vi "HRV_뽑아내기.vi"() -> ()   [LabVIEW 2014]
uses:
  <vilib>/Utility/file.llb/Read From Spreadsheet File (string).vi
  <vilib>/Utility/file.llb/Read From Spreadsheet File (I64).vi
  <vilib>/Utility/file.llb/Read From Spreadsheet File (DBL).vi
  <vilib>/Utility/file.llb/Write To Spreadsheet File (DBL).vi
panel:
  out "Array":dbl[][](array[numeric])
  in  "피험자이름":path=path "C:/Users/Jaehong/Desktop/Classifiers/HRV_EEG/ERP_total/강병훈/ERP_total.txt"
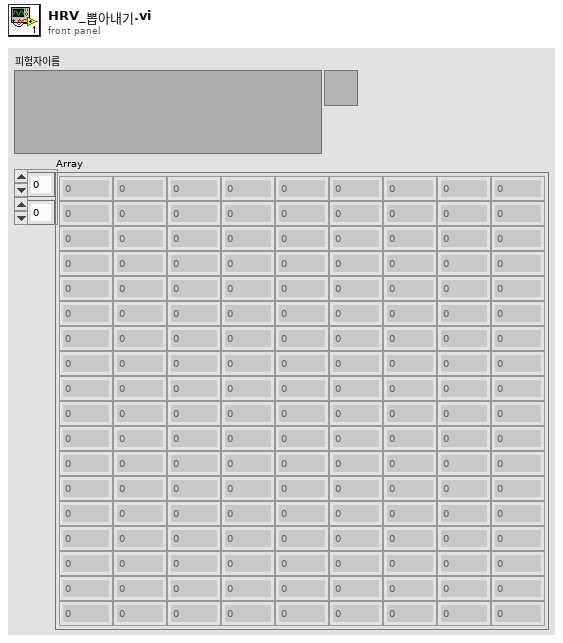
[diagram p1: front panel]
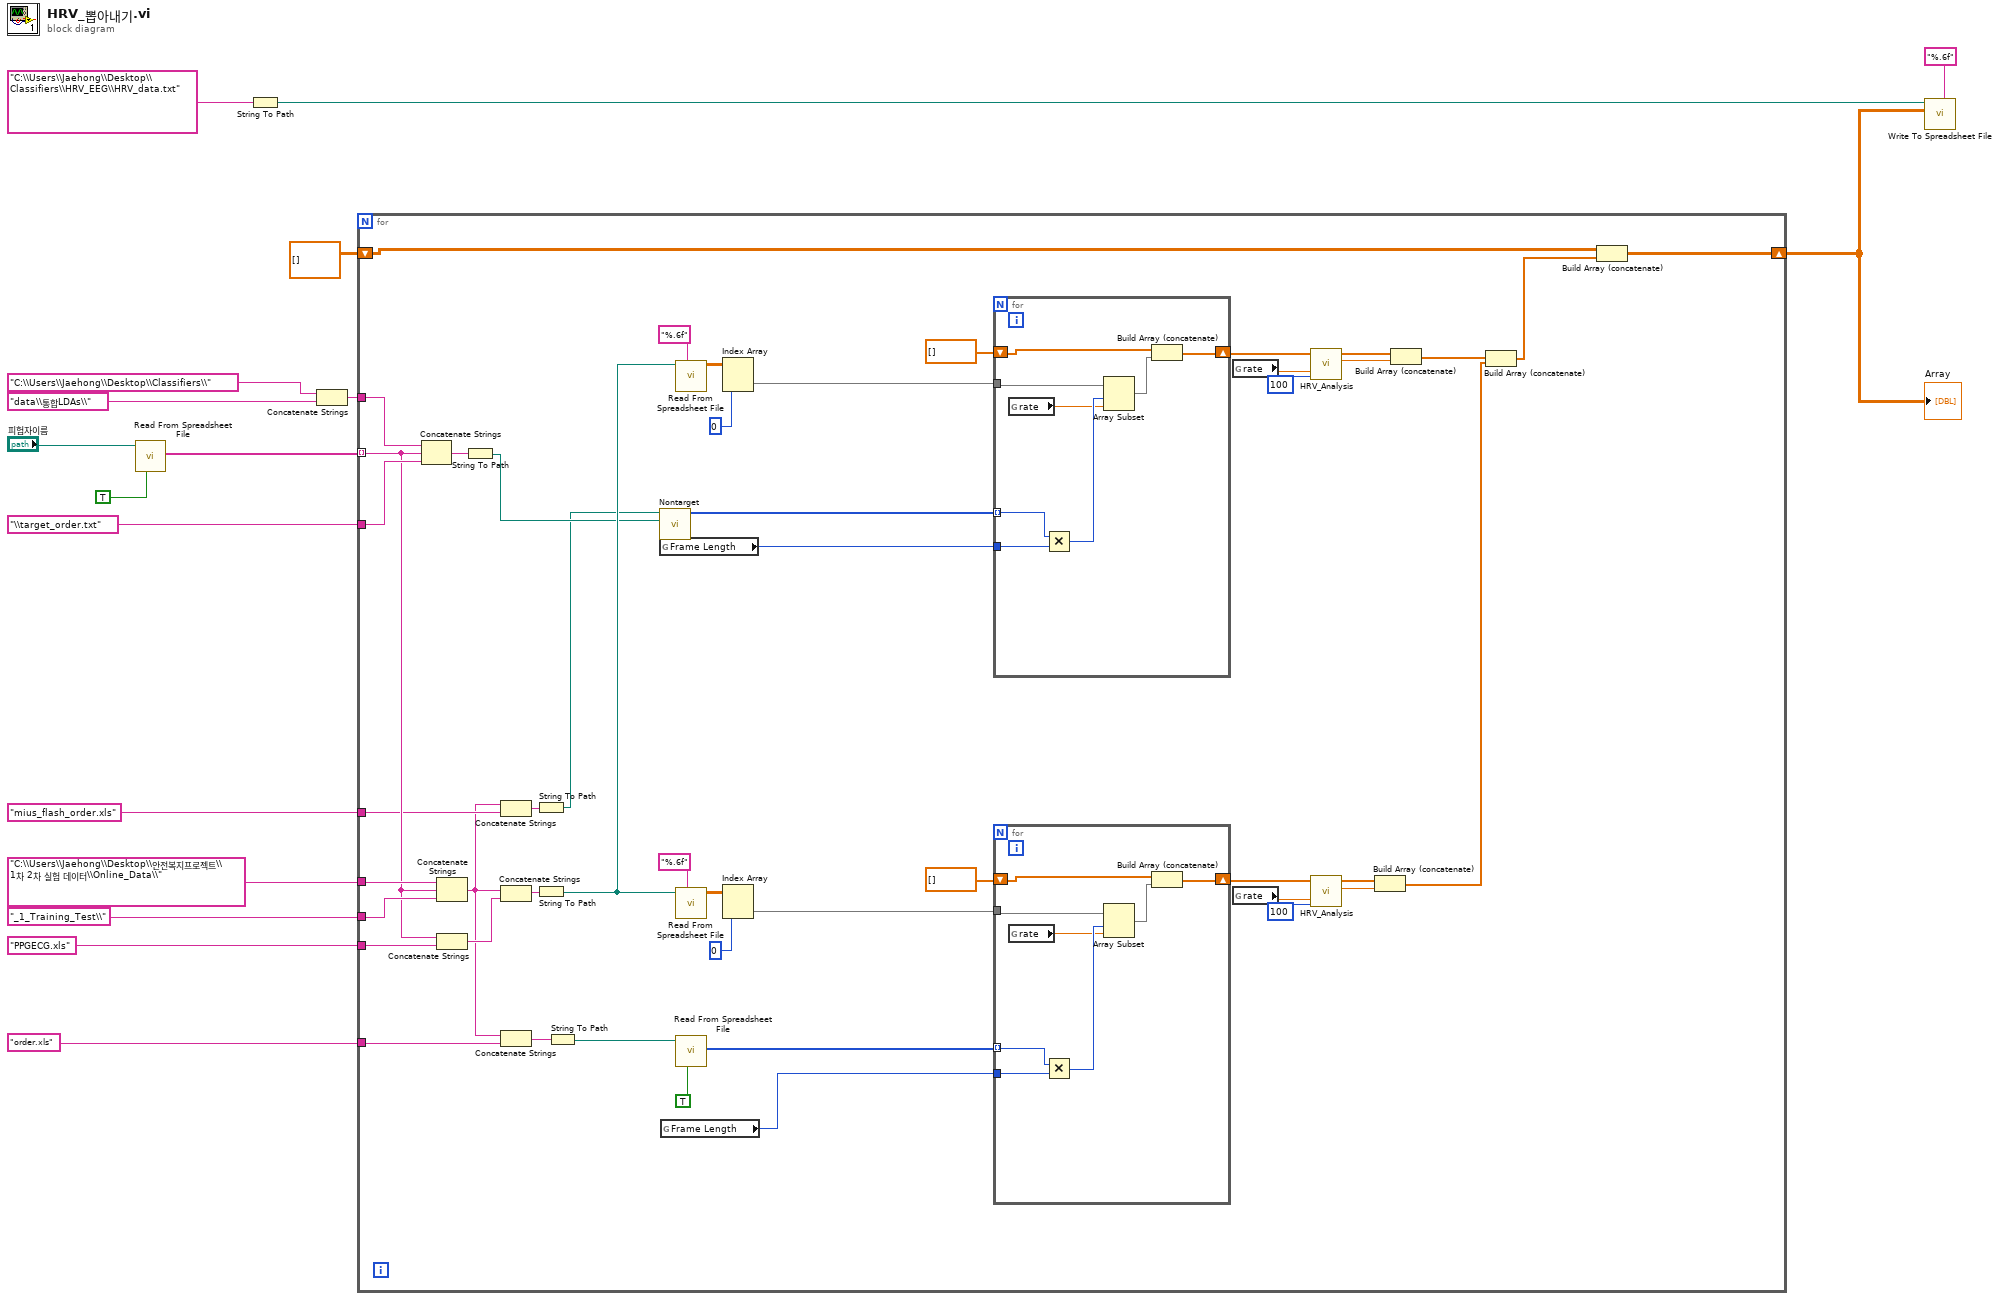
[diagram p0: block diagram]
diagram:
  n1 = call-poly <vilib>:"Read From Spreadsheet File.vi"("transpose (no:F)"=TRUE, "file path (dialog if empty)"="피험자이름") -> ("first row"=w13:string[])  [unwired: 5 in, 4 out]
  n2 = String To Path(string="C:\\Users\\Jaehong\\Desktop\\Classifiers\\HRV_EEG\\HRV_data.txt") -> (path=w2:path)
  n3 = Concatenate Strings("C:\\Users\\Jaehong\\Desktop\\Classifiers\\", "data\\통합LDAs\\") -> (w12:string)
  n4 = for {
    tunnel: w13 -> [w36] mode=indexing
    tunnel: w12 -> [w41]
    tunnel: "\\target_order.txt" -> [w40]
    tunnel: "C:\\Users\\Jaehong\\Desktop\\안전복지프로젝트\\1차 2차 실험 데이터\\Online_Data\\" -> [w39]
    tunnel: "_1_Training_Test\\" -> [w38]
    tunnel: "PPGECG.xls" -> [w37]
    tunnel: "mius_flash_order.xls" -> [w33]
    tunnel: "order.xls" -> [w29]
    shift-right: [w23] -> w3
    shift-left: dbl[][] [] -> [w22]
    n5 = Concatenate Strings(w41, w36, w40) -> (w43:string)
    n6 = Concatenate Strings(w39, w36, w38) -> (w30:string)
    n7 = Concatenate Strings(w36, w37) -> (w35:string)
    n8 = String To Path(string=w43) -> (path=w42:path)
    n9 = Concatenate Strings(w30, w33) -> (w32:string)
    n10 = Concatenate Strings(w30, w35) -> (w34:string)
    n11 = Concatenate Strings(w30, w29) -> (w28:string)
    n12 = String To Path(string=w32) -> (path=w31:path)
    n13 = String To Path(string=w34) -> (path=w44:path)
    n14 = String To Path(string=w28) -> (path=w27:path)
    n15 = call "Nontarget.vi"("Target_Total"=w42, "Mius_flash_order"=w31) -> ("Nontarget_order"=w62:i64[])  [unwired: 9 in]
    n16 = global read "Control_Panel.vi" "Frame Length"() -> (w61:i32)
    n17 = global read "Control_Panel.vi" "Frame Length"() -> (w50:i32)
    n18 = call-poly <vilib>:"Read From Spreadsheet File.vi"("format (%.3f)"="%.6f", "file path (dialog if empty)"=w44) -> ("all rows"=w64:dbl[][])  [unwired: 5 in, 4 out]
    n19 = call-poly <vilib>:"Read From Spreadsheet File.vi"("format (%.3f)"="%.6f", "file path (dialog if empty)"=w44) -> ("all rows"=w54:dbl[][])  [unwired: 5 in, 4 out]
    n20 = call-poly <vilib>:"Read From Spreadsheet File.vi"("transpose (no:F)"=TRUE, "file path (dialog if empty)"=w27) -> ("first row"=w51:i64[])  [unwired: 5 in, 4 out]
    n21 = Index Array(array=w64, index (col)=0 ("index")) -> (element=w60:dbl[])  [unwired: 1 in]
    n22 = Index Array(array=w54, index (col)=0 ("index")) -> (element=w49:dbl[])  [unwired: 1 in]
    n23 = for {
      tunnel: w62 -> [w75] mode=indexing
      tunnel: w61 -> [w81]
      tunnel: w60 -> [w80]
      shift-right: [w77] -> w56
      shift-left: dbl[] [] -> [w76]
      n24 = global read "Control_Panel.vi" "rate"() -> (w74:dbl)
      n25 = Multiply(x=w75, y=w81) -> (x*y=w79:i64)
      n26 = Array Subset(array=w80, index=w79, length=w74) -> (w78:dbl[])
      n27 = Build Array (concatenate)(w76, w78) -> (w77:dbl[])
    }
    n28 = for {
      tunnel: w51 -> [w67] mode=indexing
      tunnel: w50 -> [w73]
      tunnel: w49 -> [w72]
      shift-right: [w69] -> w45
      shift-left: dbl[] [] -> [w68]
      n29 = global read "Control_Panel.vi" "rate"() -> (w66:dbl)
      n30 = Multiply(x=w67, y=w73) -> (x*y=w71:i64)
      n31 = Array Subset(array=w72, index=w71, length=w66) -> (w70:dbl[])
      n32 = Build Array (concatenate)(w68, w70) -> (w69:dbl[])
    }
    n33 = global read "Control_Panel.vi" "rate"() -> (w57:dbl)
    n34 = global read "Control_Panel.vi" "rate"() -> (w46:dbl)
    n35 = call "HRV_Analysis.vi"("Frame Length"=100, "Sample Rate"=w57, "PPG_Data"=w56) -> ("PPI"=w20:dbl, "PRV% (VLF, LF, HF)"=w26:dbl[])  [unwired: 7 in]
    n36 = call "HRV_Analysis.vi"("Frame Length"=100, "Sample Rate"=w46, "PPG_Data"=w45) -> ("PPI"=w18:dbl, "PRV% (VLF, LF, HF)"=w25:dbl[])  [unwired: 7 in]
    n37 = Build Array (concatenate)(w25, w18) -> (w19:dbl[])
    n38 = Build Array (concatenate)(w26, w20) -> (w21:dbl[])
    n39 = Build Array (concatenate)(w21, w19) -> (w24:dbl[])
    n40 = Build Array (concatenate)(w22, w24) -> (w23:dbl[][])
  }
  "Array" <- w3
  n41 = call-poly <vilib>:"Write To Spreadsheet File.vi"("format (%.3f)"="%.6f", "2D data"=w3, "file path (dialog if empty)"=w2) -> ()  [unwired: 5 in, 1 out]
